vi "svl_Get Next Event.vi"(7 "Event Queue In":string[](array[string])) -> (2 "Next Event":string, 3 "Event Queue Out":string[](array[string]))   [LabVIEW 2017]
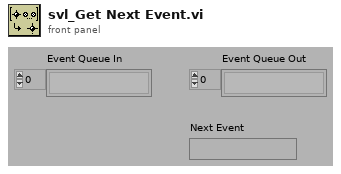
[diagram p1: front panel]
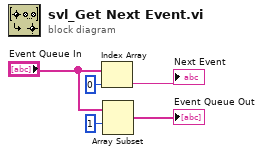
[diagram p0: block diagram]
diagram:
  n1 = Index Array(array="Event Queue In", index=0) -> (element=→"Next Event":string)
  n2 = Array Subset(array="Event Queue In", index=1) -> (→"Event Queue Out":string[])  [unwired: 1 in]
